vi "Release.vi"(8 "error in (no error)":errorcluster, 10 "Force destroy? (F)":bool, 11 "Notifier in":refnum<class "Notifier.lvclass">) -> (0 "error out":errorcluster, 2 "Last Data Notification":refnum<class "Data.lvclass">, 3 "Notifier name":string)   [LabVIEW 2020, in "Data.lvlib" / "Notifier.lvclass"]
doc: "Release the notifier."
uses:
  Notifier.lvclass
  Data.lvclass
  Notifier.lvclass/Notifier.ctl
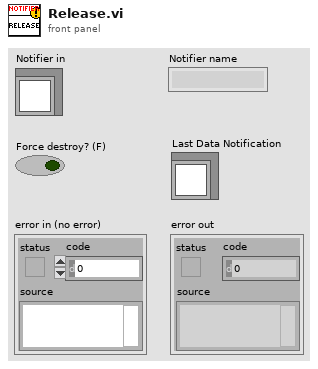
[diagram p1: front panel]
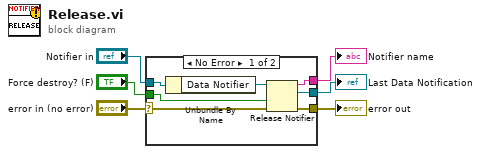
[diagram p0: block diagram]
diagram:
  n1 = case shown="No Error" "error in (no error)" {
    selector: "error in (no error)" -> [w12 w14]
    tunnel: [w11 w14] -> w5
    tunnel: "Notifier in" -> [w13 _]
    tunnel: [w10 _] -> w3
    tunnel: "Force destroy? (F)" -> [w8 _]
    tunnel: [w7 _] -> w1
    frame No Error {
      n2 = Unbundle By Name(w13) -> ("Data Notifier"=w9:refnum<notifier>)
      n3 = Release Notifier(notifier=w9, force destroy? (F)=w8, error in (no error)=w12) -> (notifier name=w7:string, last notification=w10:refnum<class "Data.lvclass">, error out=w11:errorcluster)
    }
    frame Error {
    }
  }
  "error out" <- w5
  "Last Data Notification" <- w3
  "Notifier name" <- w1
